vi "aft_Load_AFT_Fixed-Point_Settings_Sub.vi"(8 "error in (no error)":errorcluster, 11 "selected path":path) -> (0 "error out":errorcluster, 2 "AFT fixed-point settings":T1={"algorithm"=0, "filter length"=128, "step size"=0.0999985, "encoding"={"x(n) word length"=24, "x(n) integer word length"=1, "d(n) word length"=24, "d(n) integer word length"=1, "w(n) word length"=24, "w(n) integer word length"=1, "step size word length"=16, "step size integer word length"=-2}} {"algorithm" items=["LMS"]})   [LabVIEW 2017, in "NI_AdaptiveFilter.lvlib"]
doc: "Load AFT Fixed-Point Settings sub VI."
uses:
  <vilib>/addons/Adaptive Filters/NI_AdaptiveFilter.lvlib
  <vilib>/addons/Adaptive Filters/Utilities/AFT Fixed-Point Settings.ctl
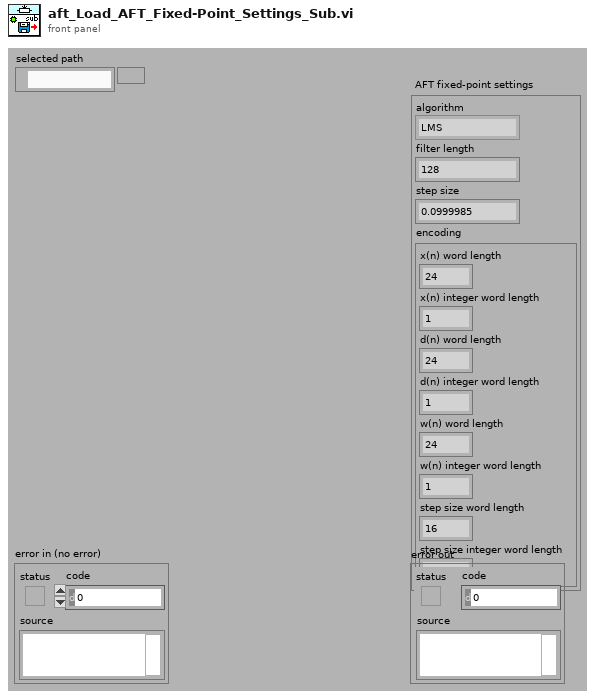
[diagram p1: front panel]
types:
  T1 = typedef "NI_AdaptiveFilter.lvlib/AFT Fixed-Point Settings.ctl" = cluster{"algorithm":u16, "filter length":i32, "step size":dbl, "encoding":cluster{"x(n) word length":i32, "x(n) integer word length":i32, "d(n) word length":i32, "d(n) integer word length":i32, "w(n) word length":i32, "w(n) integer word length":i32, "step size word length":i32, "step size integer word length":i32}}
  T2 = enum16{"open", "replace", "create", "open or create", "replace or create", "replace or create with confirmation"}
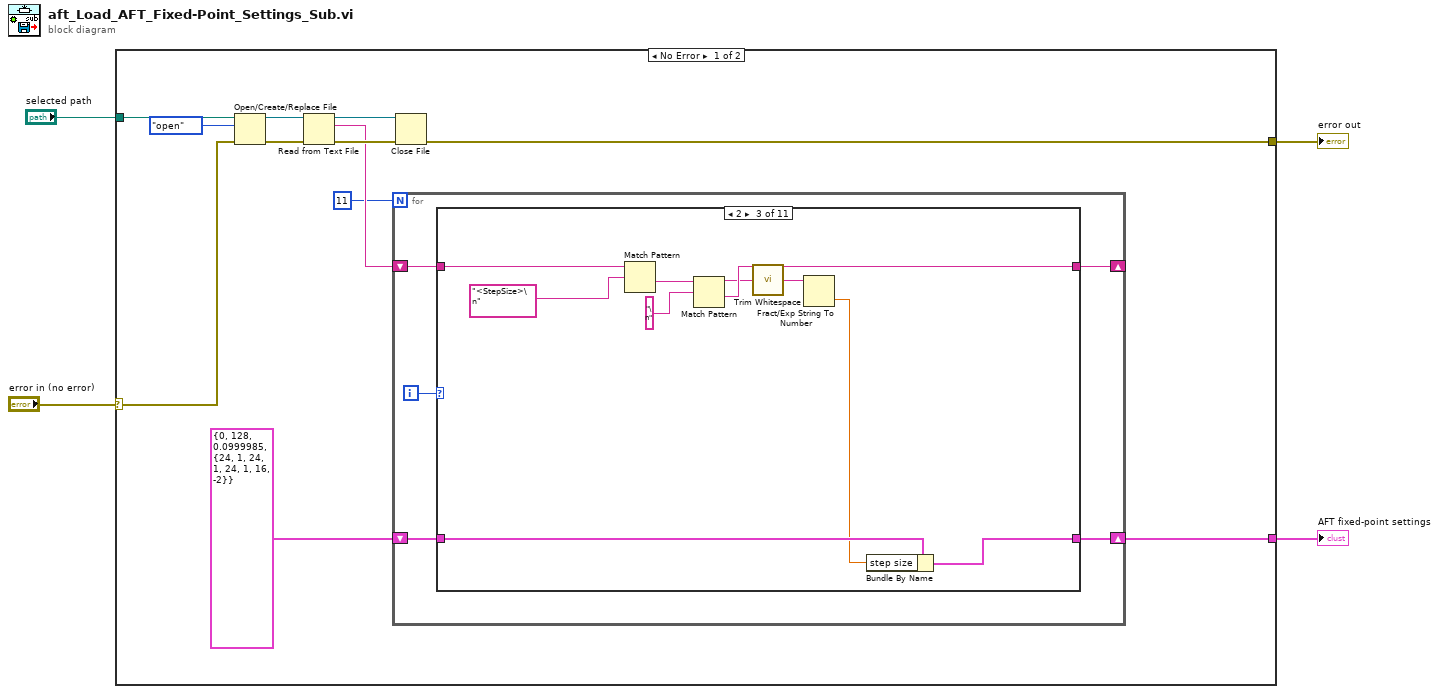
[diagram p0: block diagram]
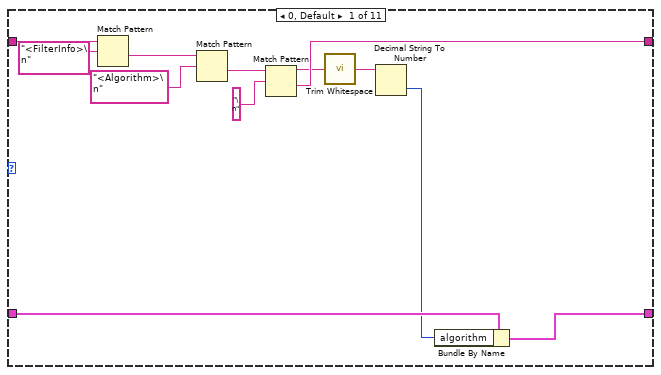
[diagram p2: hidden frame]
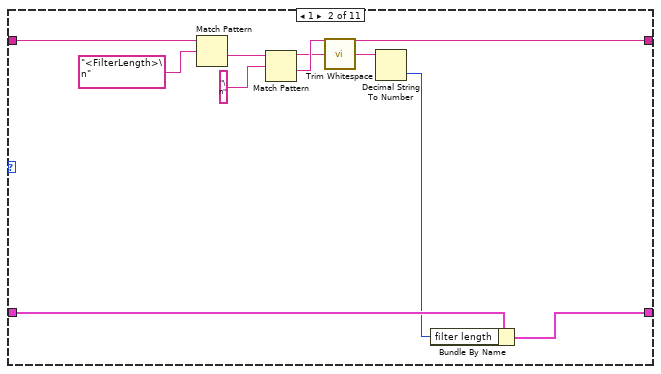
[diagram p3: hidden frame]
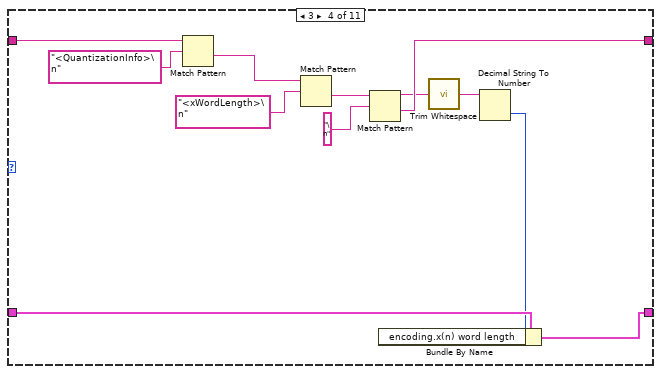
[diagram p4: hidden frame]
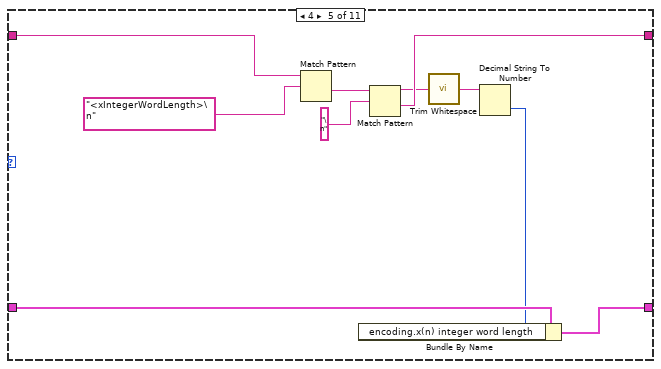
[diagram p5: hidden frame]
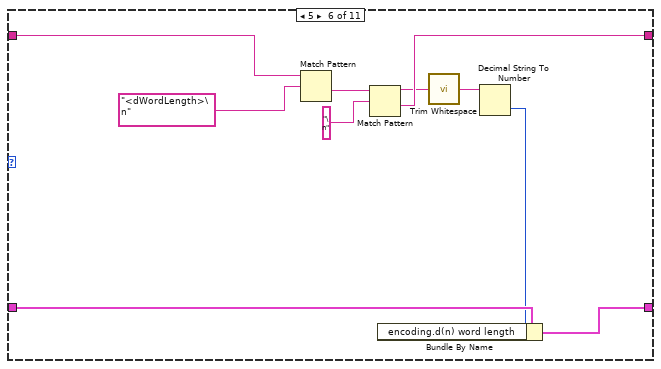
[diagram p6: hidden frame]
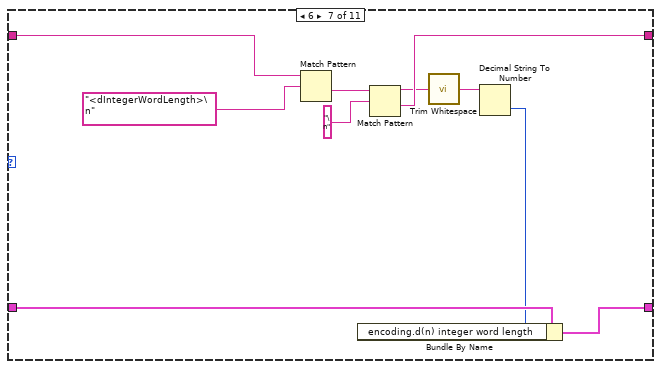
[diagram p7: hidden frame]
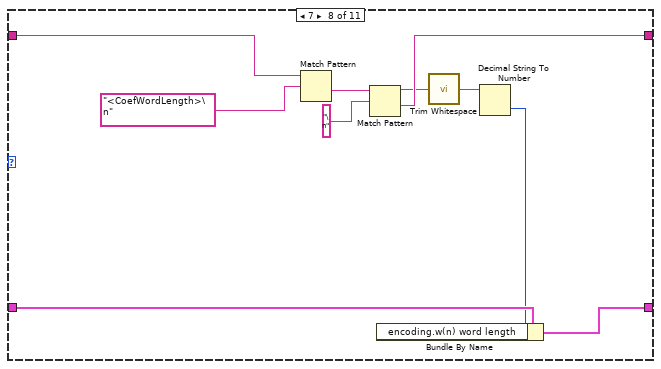
[diagram p8: hidden frame]
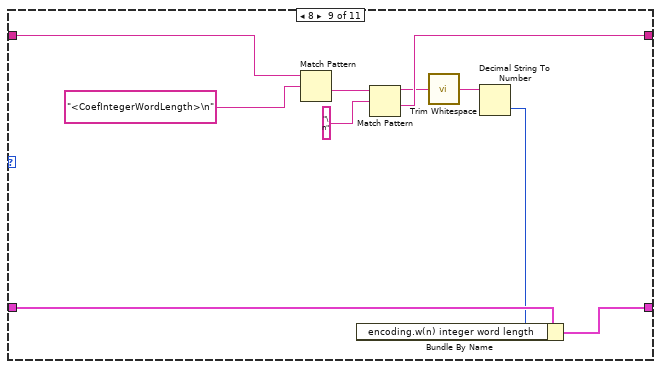
[diagram p9: hidden frame]
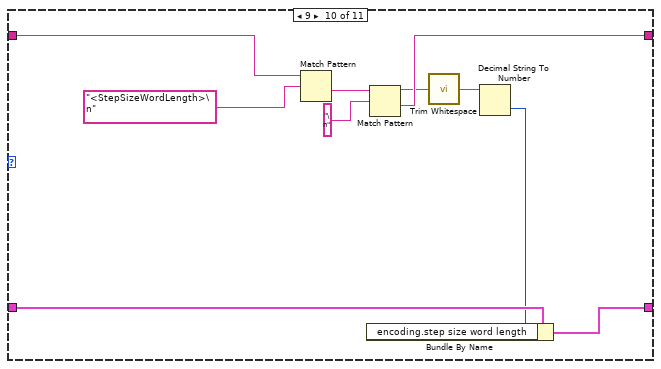
[diagram p10: hidden frame]
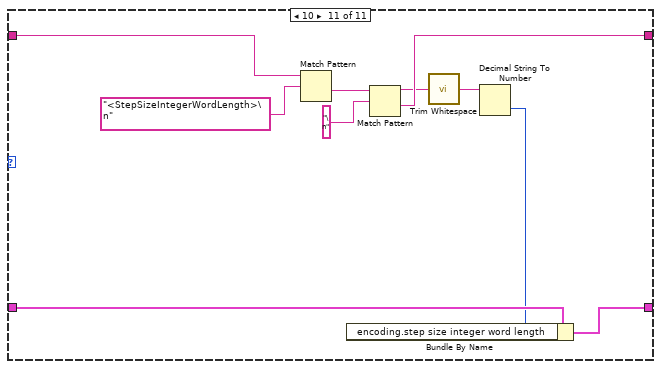
[diagram p11: hidden frame]
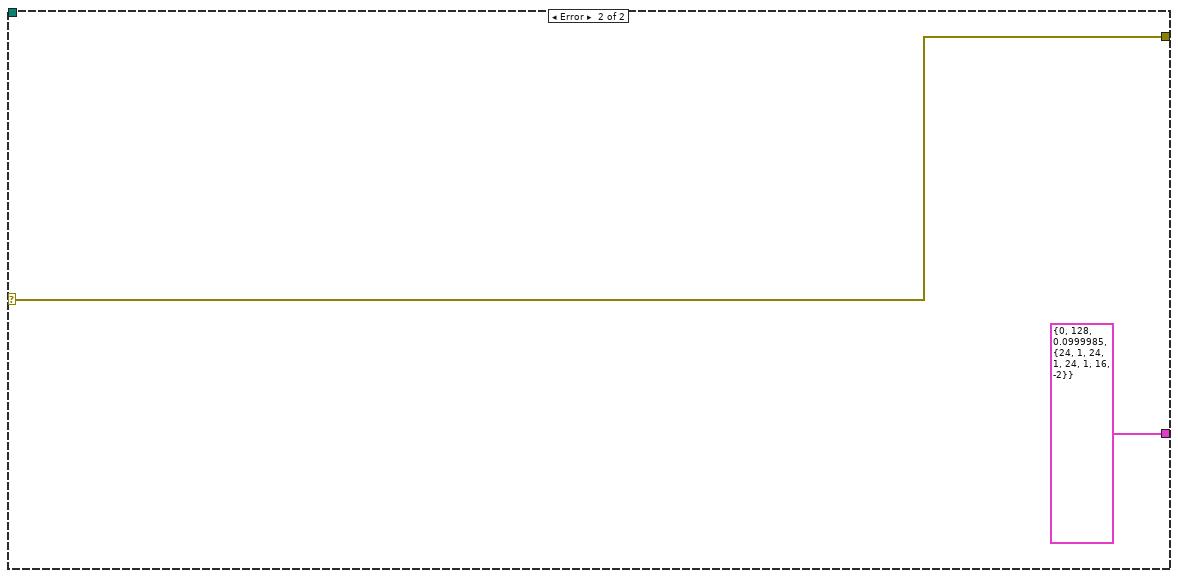
[diagram p12: hidden frame]
diagram:
  n1 = case shown="No Error" "error in (no error)" {
    selector: "error in (no error)" -> [w15 w137]
    tunnel: "selected path" -> [w16 _]
    tunnel: [w9 w137] -> w3
    tunnel: [w6 T1 {"algorithm"=0, "filter length"=128, "step size"=0.0999985, "encoding"={"x(n) word length"=24, "x(n) integer word length"=1, "d(n) word length"=24, "d(n) integer word length"=1, "w(n) word length"=24, "w(n) integer word length"=1, "step size word length"=16, "step size integer word length"=-2}} ("AFT fixed-point settings 2")] -> w1
    frame No Error {
      n2 = Open/Create/Replace File(file path (use dialog)=w16, error in=w15, operation (0:open)=T2."open") -> (refnum out=w13:refnum<file>, error out=w12:errorcluster)  [unwired: 4 out]
      n3 = Read from Text File(file (use dialog)=w13, error in=w12) -> (refnum out=w11:refnum<file>, text=w8:string, error out=w10:errorcluster)  [unwired: 3 out]
      n4 = for {
        N: 11 -> [_]
        shift-right: [w19] -> _
        shift-left: w8 -> [w20]
        shift-right: [w17] -> w6
        shift-left: T1 {"algorithm"=0, "filter length"=128, "step size"=0.0999985, "encoding"={"x(n) word length"=24, "x(n) integer word length"=1, "d(n) word length"=24, "d(n) integer word length"=1, "w(n) word length"=24, "w(n) integer word length"=1, "step size word length"=16, "step size integer word length"=-2}} ("AFT fixed-point settings 2") -> [w18]
        i -> [w21]
        n5 = case shown="2" w21 {
          tunnel: w20 -> [w33 w36 w46 w59 w68 w78 w88 w98 w108 w118 w128]
          tunnel: [w29 w42 w52 w64 w74 w84 w94 w104 w114 w124 w134] -> w19
          tunnel: w18 -> [w26 w39 w49 w61 w71 w81 w91 w101 w111 w121 w131]
          tunnel: [w24 w37 w47 w58 w69 w79 w89 w99 w109 w119 w129] -> w17
          frame 0, Default {
            n6 = Match Pattern(string=w33, regular expression="<FilterInfo>\n") -> (after substring=w31:string)  [unwired: 4 out]
            n7 = Match Pattern(string=w31, regular expression="<Algorithm>\n" ("key")) -> (after substring=w30:string)  [unwired: 4 out]
            n8 = Match Pattern(string=w30, regular expression="\n") -> (before substring=w28:string, after substring=w29:string)  [unwired: 3 out]
            n9 = call <vilib>:"Trim Whitespace.vi"("string"=w28) -> ("trimmed string"=w27:string)  [unwired: 1 in]
            n10 = Decimal String To Number(string=w27) -> (number=w25:i32)  [unwired: 3 out]
            n11 = Bundle By Name(cluster=w26, "algorithm"=w25) -> (w24:T1)
          }
          frame 1 {
            n12 = Match Pattern(string=w36, regular expression="<FilterLength>\n" ("key")) -> (after substring=w43:string)  [unwired: 4 out]
            n13 = Match Pattern(string=w43, regular expression="\n") -> (before substring=w41:string, after substring=w42:string)  [unwired: 3 out]
            n14 = call <vilib>:"Trim Whitespace.vi"("string"=w41) -> ("trimmed string"=w40:string)  [unwired: 1 in]
            n15 = Decimal String To Number(string=w40) -> (number=w38:i32)  [unwired: 3 out]
            n16 = Bundle By Name(cluster=w39, "filter length"=w38) -> (w37:T1)
          }
          frame 2 {
            n17 = Match Pattern(string=w46, regular expression="<StepSize>\n" ("key")) -> (after substring=w53:string)  [unwired: 4 out]
            n18 = Match Pattern(string=w53, regular expression="\n") -> (before substring=w51:string, after substring=w52:string)  [unwired: 3 out]
            n19 = call <vilib>:"Trim Whitespace.vi"("string"=w51) -> ("trimmed string"=w50:string)  [unwired: 1 in]
            n20 = Fract/Exp String To Number(string=w50) -> (number=w48:dbl)  [unwired: 4 out]
            n21 = Bundle By Name(cluster=w49, "step size"=w48) -> (w47:T1)
          }
          frame 3 {
            n22 = Match Pattern(string=w59, regular expression="<QuantizationInfo>\n" ("key")) -> (after substring=w57:string)  [unwired: 4 out]
            n23 = Match Pattern(string=w57, regular expression="<xWordLength>\n" ("key")) -> (after substring=w65:string)  [unwired: 4 out]
            n24 = Match Pattern(string=w65, regular expression="\n") -> (before substring=w63:string, after substring=w64:string)  [unwired: 3 out]
            n25 = call <vilib>:"Trim Whitespace.vi"("string"=w63) -> ("trimmed string"=w62:string)  [unwired: 1 in]
            n26 = Decimal String To Number(string=w62) -> (number=w60:i32)  [unwired: 3 out]
            n27 = Bundle By Name(cluster=w61, "encoding.x(n) word length"=w60) -> (w58:T1)
          }
          frame 4 {
            n28 = Match Pattern(string=w68, regular expression="<xIntegerWordLength>\n" ("key")) -> (after substring=w75:string)  [unwired: 4 out]
            n29 = Match Pattern(string=w75, regular expression="\n") -> (before substring=w73:string, after substring=w74:string)  [unwired: 3 out]
            n30 = call <vilib>:"Trim Whitespace.vi"("string"=w73) -> ("trimmed string"=w72:string)  [unwired: 1 in]
            n31 = Decimal String To Number(string=w72) -> (number=w70:i32)  [unwired: 3 out]
            n32 = Bundle By Name(cluster=w71, "encoding.x(n) integer word length"=w70) -> (w69:T1)
          }
          frame 5 {
            n33 = Match Pattern(string=w78, regular expression="<dWordLength>\n" ("key")) -> (after substring=w85:string)  [unwired: 4 out]
            n34 = Match Pattern(string=w85, regular expression="\n") -> (before substring=w83:string, after substring=w84:string)  [unwired: 3 out]
            n35 = call <vilib>:"Trim Whitespace.vi"("string"=w83) -> ("trimmed string"=w82:string)  [unwired: 1 in]
            n36 = Decimal String To Number(string=w82) -> (number=w80:i32)  [unwired: 3 out]
            n37 = Bundle By Name(cluster=w81, "encoding.d(n) word length"=w80) -> (w79:T1)
          }
          frame 6 {
            n38 = Match Pattern(string=w88, regular expression="<dIntegerWordLength>\n" ("key")) -> (after substring=w95:string)  [unwired: 4 out]
            n39 = Match Pattern(string=w95, regular expression="\n") -> (before substring=w93:string, after substring=w94:string)  [unwired: 3 out]
            n40 = call <vilib>:"Trim Whitespace.vi"("string"=w93) -> ("trimmed string"=w92:string)  [unwired: 1 in]
            n41 = Decimal String To Number(string=w92) -> (number=w90:i32)  [unwired: 3 out]
            n42 = Bundle By Name(cluster=w91, "encoding.d(n) integer word length"=w90) -> (w89:T1)
          }
          frame 7 {
            n43 = Match Pattern(string=w98, regular expression="<CoefWordLength>\n" ("key")) -> (after substring=w105:string)  [unwired: 4 out]
            n44 = Match Pattern(string=w105, regular expression="\n") -> (before substring=w103:string, after substring=w104:string)  [unwired: 3 out]
            n45 = call <vilib>:"Trim Whitespace.vi"("string"=w103) -> ("trimmed string"=w102:string)  [unwired: 1 in]
            n46 = Decimal String To Number(string=w102) -> (number=w100:i32)  [unwired: 3 out]
            n47 = Bundle By Name(cluster=w101, "encoding.w(n) word length"=w100) -> (w99:T1)
          }
          frame 8 {
            n48 = Match Pattern(string=w108, regular expression="<CoefIntegerWordLength>\n" ("key")) -> (after substring=w115:string)  [unwired: 4 out]
            n49 = Match Pattern(string=w115, regular expression="\n") -> (before substring=w113:string, after substring=w114:string)  [unwired: 3 out]
            n50 = call <vilib>:"Trim Whitespace.vi"("string"=w113) -> ("trimmed string"=w112:string)  [unwired: 1 in]
            n51 = Decimal String To Number(string=w112) -> (number=w110:i32)  [unwired: 3 out]
            n52 = Bundle By Name(cluster=w111, "encoding.w(n) integer word length"=w110) -> (w109:T1)
          }
          frame 9 {
            n53 = Match Pattern(string=w118, regular expression="<StepSizeWordLength>\n" ("key")) -> (after substring=w125:string)  [unwired: 4 out]
            n54 = Match Pattern(string=w125, regular expression="\n") -> (before substring=w123:string, after substring=w124:string)  [unwired: 3 out]
            n55 = call <vilib>:"Trim Whitespace.vi"("string"=w123) -> ("trimmed string"=w122:string)  [unwired: 1 in]
            n56 = Decimal String To Number(string=w122) -> (number=w120:i32)  [unwired: 3 out]
            n57 = Bundle By Name(cluster=w121, "encoding.step size word length"=w120) -> (w119:T1)
          }
          frame 10 {
            n58 = Match Pattern(string=w128, regular expression="<StepSizeIntegerWordLength>\n" ("key")) -> (after substring=w135:string)  [unwired: 4 out]
            n59 = Match Pattern(string=w135, regular expression="\n") -> (before substring=w133:string, after substring=w134:string)  [unwired: 3 out]
            n60 = call <vilib>:"Trim Whitespace.vi"("string"=w133) -> ("trimmed string"=w132:string)  [unwired: 1 in]
            n61 = Decimal String To Number(string=w132) -> (number=w130:i32)  [unwired: 3 out]
            n62 = Bundle By Name(cluster=w131, "encoding.step size integer word length"=w130) -> (w129:T1)
          }
        }
      }
      n63 = Close File(refnum=w11, error in=w10) -> (error out=w9:errorcluster)  [unwired: 1 out]
    }
    frame Error {
    }
  }
  "AFT fixed-point settings" <- w1
  "error out" <- w3
